vi "Car Wash Main.vi"(0 "Deluxe Wash":bool, 7 "Economy wash":bool, 9 "stop":bool, 11 "Error in":errorcluster) -> (4 "Under body wash":bool, 6 "Soap application":bool, 8 "Main high pressure wash":bool, 10 "Clear water rinse":bool, 15 "error out":errorcluster)   [LabVIEW 2020, in "Car Wash.lvlib"]
doc: "This system is a state machine of car wash system which has two different modes for users such as premium and genric car wash"
uses:
  Car Wash.lvlib
  Typedefs/Queue operations.ctl
  Typedefs/Car wash data.ctl
panel:
  out "Elapsed Time":dbl
  out "Vehicle out of position":bool
  out "Air dry":bool
  in  "Air dry\nposition\nswitch":bool
  in  "Main wash\nPosition \nswitch":bool
  in  "Under Body\nWash Position \nswitch":bool
  # "Purchase Section"
  # "Car Wash Simulators"
  # "Car Wash Simulation Switches"
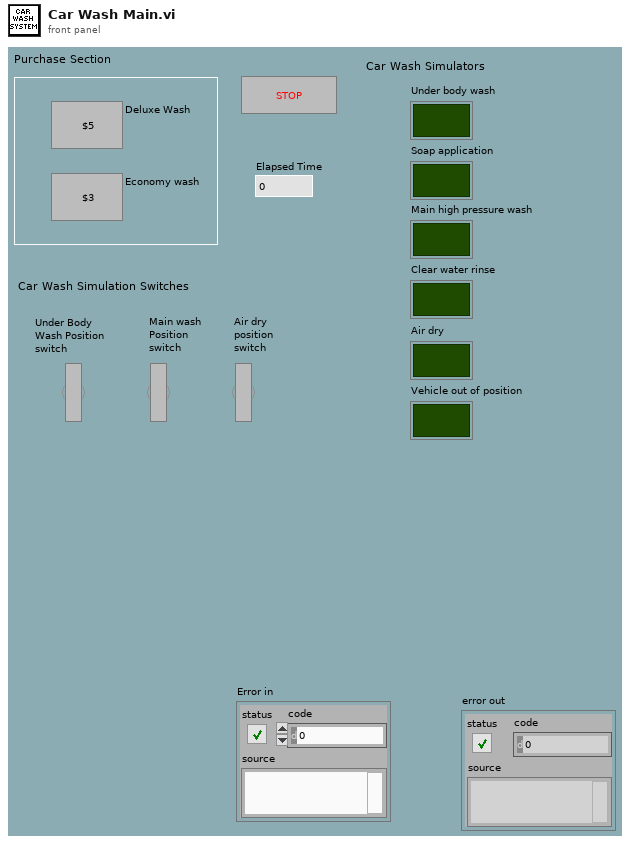
[diagram p1: front panel]
types:
  T1 = typedef "Car wash data.ctl" = cluster{"Start Time":timestamp, "Elapsed Time":dbl, "Set Time":dbl, "Previous Time":dbl, "Started?":bool, "Paused?":bool, "Enable controls ref":refnum<vi>[], "Disable controls ref":refnum<vi>[], "Soap application":bool, "Main high pressure wash":bool, "Under body wash":bool, "Clean water wash":bool, "Air dry":bool, "Vehicle out of position":bool, "Deluxe":bool, "Economy":bool, "Stop":bool}
  T2 = typedef "Car Wash.lvlib/Queue operations.ctl" = enum16{"Create queue", "Enqueue", "Enstack", "Dequeue", "Flush queue", "Release queue"}
  T3 = enum8{"Enabled", "Disabled", "Disabled and Grayed Out"}
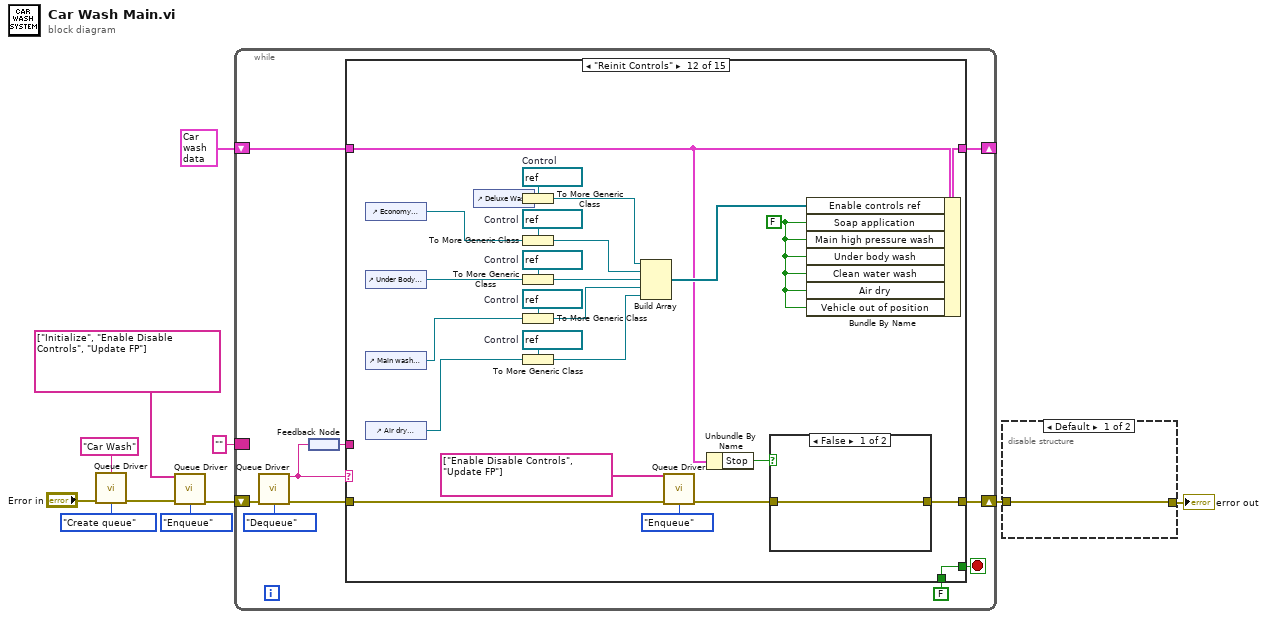
[diagram p0: block diagram]
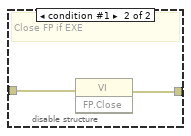
[diagram p2: hidden frame]
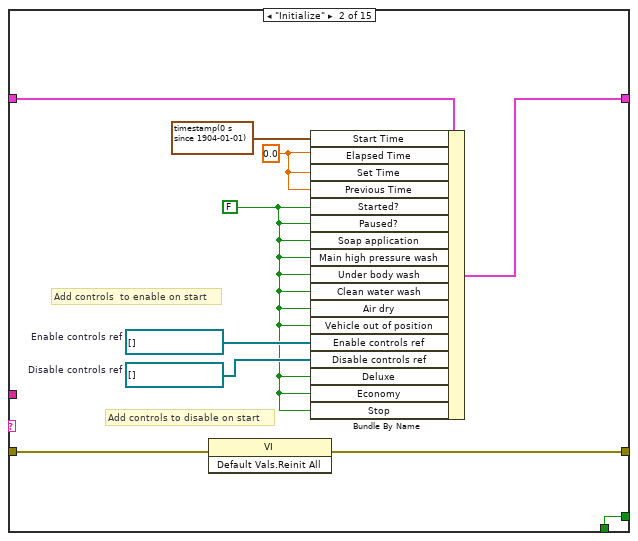
[diagram p4: hidden frame]
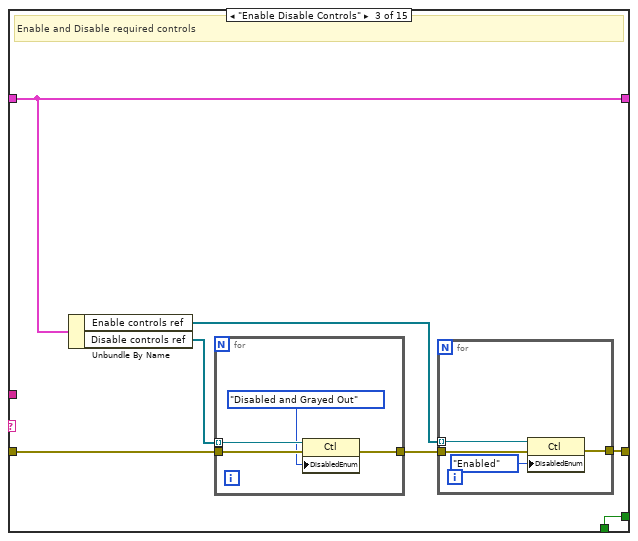
[diagram p5: hidden frame]
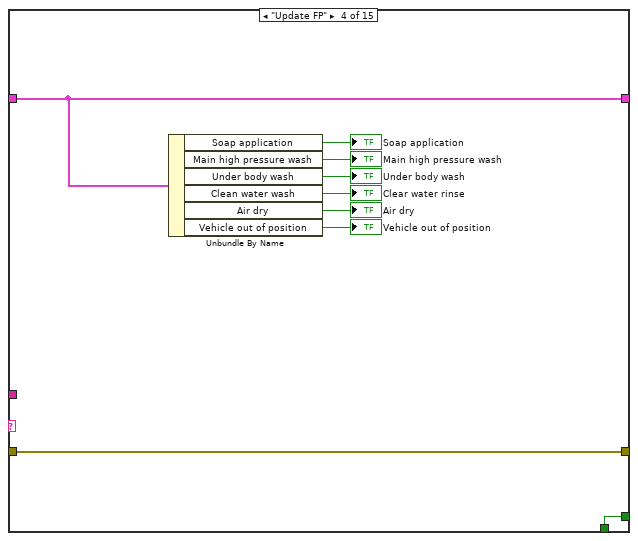
[diagram p6: hidden frame]
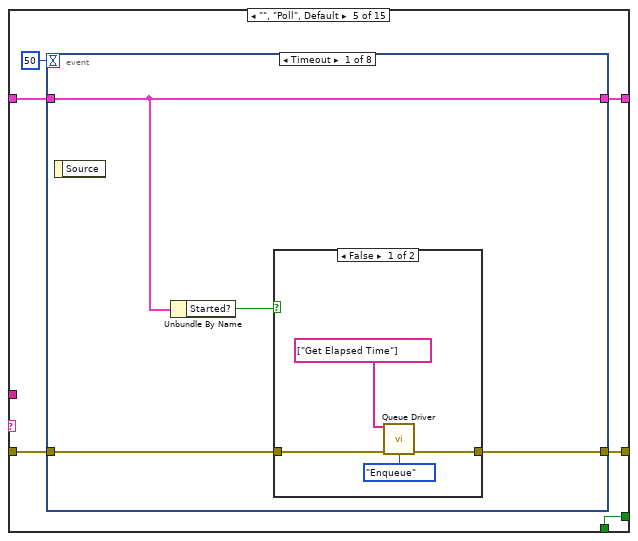
[diagram p7: hidden frame]
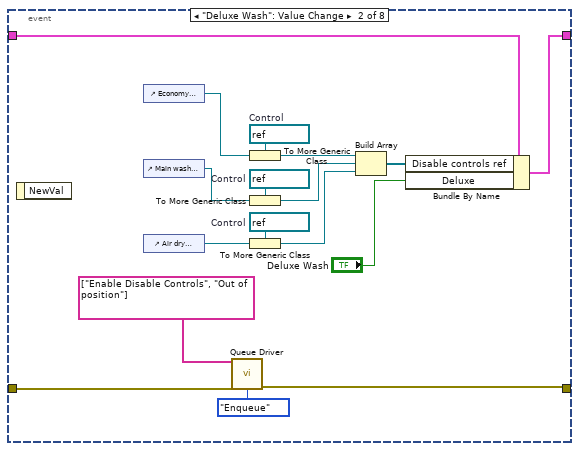
[diagram p9: hidden frame]
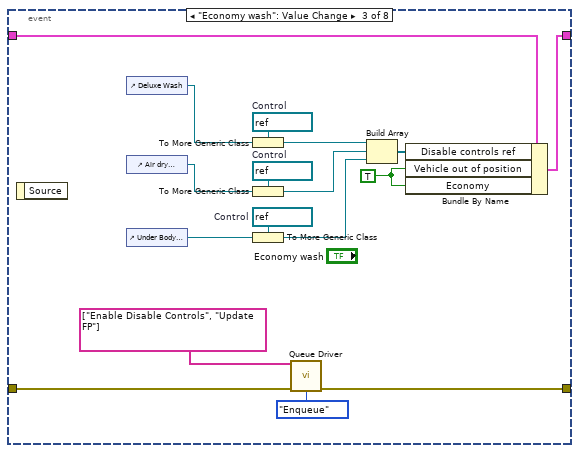
[diagram p10: hidden frame]
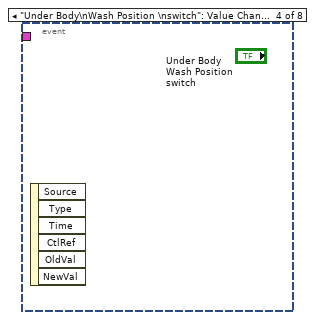
[diagram p11: hidden frame]
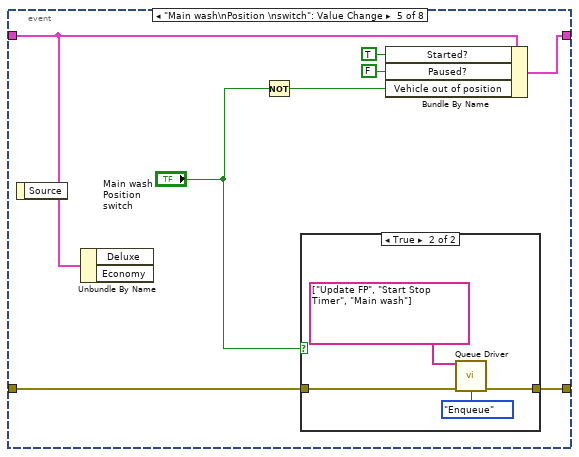
[diagram p12: hidden frame]
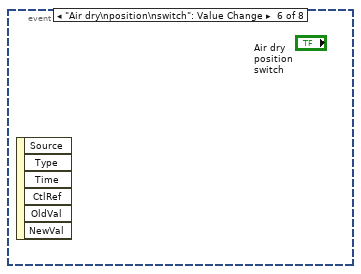
[diagram p14: hidden frame]
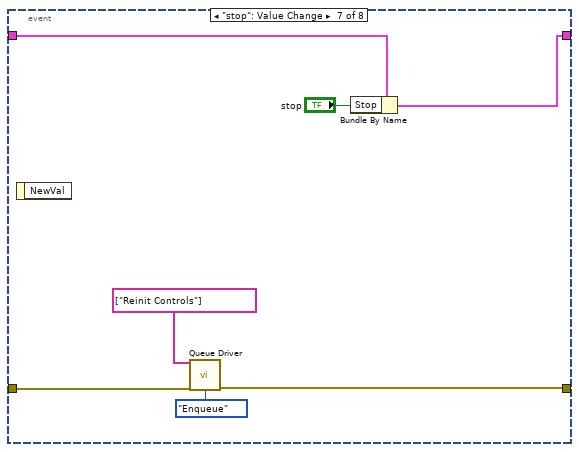
[diagram p15: hidden frame]
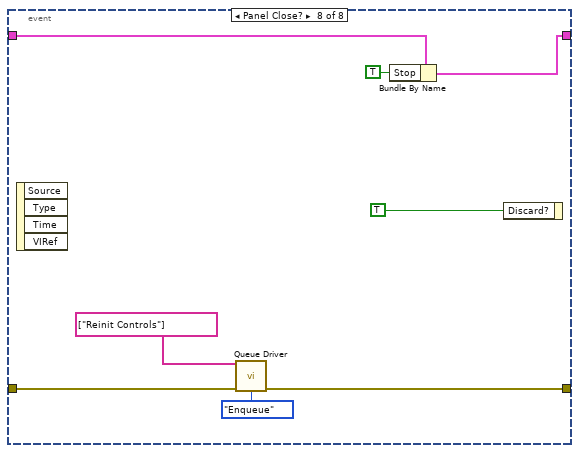
[diagram p16: hidden frame]
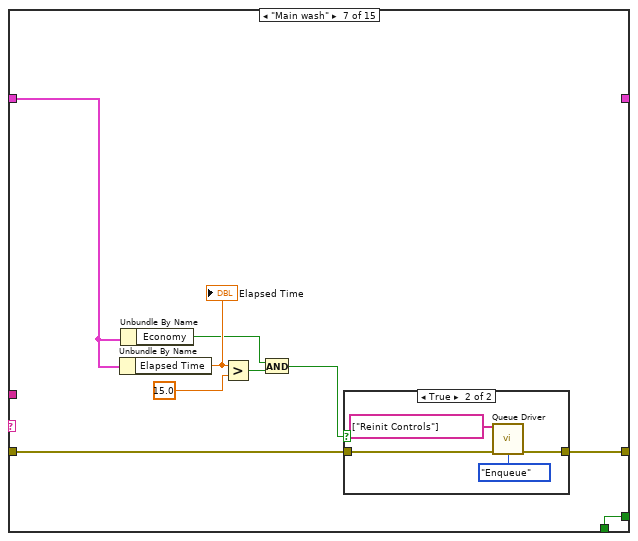
[diagram p18: hidden frame]
diagram:
  n1 = call "Queue Driver.vi"("Name"="Car Wash", "Error in"="Error in", "Operation"=Queue_operations."Create queue") -> ("Error out"=w10:errorcluster)  [unwired: 11 in, 1 out]
  n2 = call "Queue Driver.vi"("States"=string[] ["Initialize", "Enable Disable Controls", "Update FP"], "Error in"=w10, "Operation"=Queue_operations."Enqueue") -> ("Error out"=w5:errorcluster)  [unwired: 11 in, 1 out]
  n3 = while {
    border: "" ("Dequeued State") -> [_]
    shift-right: [w16] -> w3
    shift-left: w5 -> [w21]
    shift-right: [w14] -> _
    shift-left: T1 {"Start Time"=timestamp(0 s since 1904-01-01), "Elapsed Time"=0.0, "Set Time"=0.0, "Previous Time"=0.0, "Started?"=FALSE, "Paused?"=FALSE, "Enable controls ref"=[], "Disable controls ref"=[], "Soap application"=FALSE, "Main high pressure wash"=FALSE, "Under body wash"=FALSE, "Clean water wash"=FALSE, "Air dry"=FALSE, "Vehicle out of position"=FALSE, "Deluxe"=FALSE, "Economy"=FALSE, "Stop"=FALSE} -> [w15]
    stop <- w12 stop-if-true
    n4 = call "Queue Driver.vi"("Error in"=w21, "Operation"=Queue_operations."Dequeue") -> ("Dequeued State"=w19:string, "Error out"=w17:errorcluster)  [unwired: 12 in]
    n5 = feedback-in #1(w19) -> ()
    n6 = feedback #1() -> (w18:string)
    n7 = case shown="\"Reinit Controls\"" w19 {
      tunnel: w18 -> [_ _ _ _ _ _ _ _ _ _ _ _ _ w230 _]
      tunnel: [w23 w29 w37 w50 w60 w136 w139 w152 w154 w159 w164 w175 w204 w227 w249] -> w16
      tunnel: w17 -> [w23 w30 w39 w50 w61 w136 w140 w152 w154 w159 w164 w185 w205 w231 w247]
      tunnel: w15 -> [w24 w34 w41 w58 w62 _ w142 _ _ w157 w167 w174 w210 w226 w246]
      tunnel: [w24 w31 w41 w58 w63 _ _ _ _ w161 w166 w178 w209 w226 w246] -> w14
      tunnel: FALSE -> [w22 w26 w35 w51 w59 w137 w146 w153 w155 w160 w165 w184 w203 w225 _]
      tunnel: [w22 w26 w35 w51 w59 w137 w146 w153 w155 w160 w165 w184 w203 w225 TRUE] -> w12
      frame "/***Initialize***/" {
      }
      frame "Initialize" {
        w27 = refnum<vi>[] []  # Disable controls ref
        w28 = refnum<vi>[] []  # Enable controls ref
        w25 = FALSE
        w32 = 0.0
        # "Add controls to disable on start"
        # "Add controls  to enable on start"
        n8 = invoke class="VI" method="Default Vals.Reinit All"(error in=w30) -> (error out=w29:errorcluster)  [unwired: 2 in, 2 out]
        n9 = Bundle By Name(cluster=w34, "Start Time"=timestamp(0 s since 1904-01-01), "Elapsed Time"=w32, "Set Time"=w32, "Previous Time"=w32, "Started?"=w25, "Paused?"=w25, "Soap application"=w25, "Main high pressure wash"=w25, "Under body wash"=w25, "Clean water wash"=w25, "Air dry"=w25, "Vehicle out of position"=w25, "Enable controls ref"=w28, "Disable controls ref"=w27, "Deluxe"=w25, "Economy"=w25, "Stop"=w25) -> (w31:T1)
      }
      frame "Enable Disable Controls" {
        # "Enable and Disable required controls"
        n10 = Unbundle By Name(w41) -> ("Enable controls ref"=w40:refnum<vi>[], "Disable controls ref"=w36:refnum<vi>[])
        n11 = for {
          tunnel: w39 -> [w49]
          tunnel: [w48] -> w38
          tunnel: w36 -> [w47] mode=indexing
          n12 = property class="Ctl"(reference=w47, error in=w49, "DisabledEnum"=T3."Disabled and Grayed Out" ("Disabled")) -> (error out=w48:errorcluster)  [unwired: 1 out]
        }
        n13 = for {
          tunnel: w40 -> [w45] mode=indexing
          tunnel: w38 -> [w44]
          tunnel: [w42] -> w37
          n14 = property class="Ctl"(reference=w45, error in=w44, "DisabledEnum"=T3."Enabled" ("Disabled")) -> (error out=w42:errorcluster)  [unwired: 1 out]
        }
      }
      frame "Update FP" {
        n15 = Unbundle By Name(w58) -> ("Soap application"=→"Soap application":bool, "Main high pressure wash"=→"Main high pressure wash":bool, "Under body wash"=→"Under body wash":bool, "Clean water wash"=→"Clear water rinse":bool, "Air dry"=→"Air dry":bool, "Vehicle out of position"=→"Vehicle out of position":bool)
      }
      frame "", "Poll", Default {
        n16 = event shown="[0] Timeout" {
          selector: _ -> [_ _ _ _ _ _ _ _]
          dyn-events: _ -> [_ _ _ _ _ _ _ _]
          timeout: 50 -> [_ _ _ _ _ _ _ _]
          tunnel: [w68 w89 w106 _ w112 _ w122 w129] -> w63
          tunnel: w62 -> [w68 w90 w107 _ w113 _ w123 w130]
          tunnel: w61 -> [w67 w87 w102 _ w115 _ w127 w132]
          tunnel: [w66 w86 w101 _ w114 _ w126 w131] -> w60
          event Timeout {
            n17 = event-data() -> ()  [unwired: 1 in, 1 out]
            n18 = Unbundle By Name(w68) -> ("Started?"=w65:bool)
            n19 = case shown="False" w65 {
              tunnel: w67 -> [w72 w73]
              tunnel: [w71 w73] -> w66
              frame False {
                n20 = call "Queue Driver.vi"("States"=string[] ["Get Elapsed Time"], "Error in"=w72, "Operation"=Queue_operations."Enqueue") -> ("Error out"=w71:errorcluster)  [unwired: 11 in, 1 out]
              }
              frame True {
              }
            }
          }
          event "Deluxe Wash": Value Change {
            w79 = refnum<vi> refnum  # Control
            w80 = refnum<vi> refnum  # Control
            w82 = refnum<vi> refnum  # Control
            n21 = event-data() -> ()  [unwired: 1 in, 1 out]
            n22 = control-ref of="Economy wash"() -> (w83:refnum<vi>)
            n23 = control-ref of="Main wash\nPosition \nswitch"() -> (w77:refnum<vi>)
            n24 = control-ref of="Air dry\nposition\nswitch"() -> (w78:refnum<vi>)
            n25 = call "Queue Driver.vi"("States"=string[] ["Enable Disable Controls", "Out of position"], "Error in"=w87, "Operation"=Queue_operations."Enqueue") -> ("Error out"=w86:errorcluster)  [unwired: 11 in, 1 out]
            n26 = To More Generic Class(target class=w82, reference=w83) -> (generic class reference=w81:refnum<vi>)
            n27 = To More Generic Class(target class=w80, reference=w77) -> (generic class reference=w76:refnum<vi>)
            n28 = To More Generic Class(target class=w79, reference=w78) -> (generic class reference=w75:refnum<vi>)
            n29 = Build Array(w81, w76, w75) -> (w88:refnum<vi>[])
            n30 = Bundle By Name(cluster=w90, "Disable controls ref"=w88, "Deluxe"="Deluxe Wash") -> (w89:T1)
          }
          event "Economy wash": Value Change {
            w91 = TRUE ("Vehicle out of position")
            w96 = refnum<vi> refnum  # Control
            w97 = refnum<vi> refnum  # Control
            w98 = refnum<vi> refnum  # Control
            n31 = event-data() -> ()  [unwired: 1 in, 1 out]
            n32 = control-ref of="Deluxe Wash"() -> (w104:refnum<vi>)
            n33 = control-ref of="Air dry\nposition\nswitch"() -> (w92:refnum<vi>)
            n34 = control-ref of="Under Body\nWash Position \nswitch"() -> (w95:refnum<vi>)
            n35 = To More Generic Class(target class=w98, reference=w104) -> (generic class reference=w99:refnum<vi>)
            n36 = To More Generic Class(target class=w97, reference=w92) -> (generic class reference=w94:refnum<vi>)
            n37 = To More Generic Class(target class=w96, reference=w95) -> (generic class reference=w93:refnum<vi>)
            n38 = call "Queue Driver.vi"("States"=string[] ["Enable Disable Controls", "Update FP"], "Error in"=w102, "Operation"=Queue_operations."Enqueue") -> ("Error out"=w101:errorcluster)  [unwired: 11 in, 1 out]
            n39 = Build Array(w99, w94, w93) -> (w105:refnum<vi>[])
            n40 = Bundle By Name(cluster=w107, "Disable controls ref"=w105, "Vehicle out of position"=w91, "Economy"=w91) -> (w106:T1)
          }
          event "Under Body\nWash Position \nswitch": Value Change {
            n41 = event-data() -> ()  [unwired: 1 in, 6 out]
          }
          event "Main wash\nPosition \nswitch": Value Change {
            n42 = event-data() -> ()  [unwired: 1 in, 1 out]
            n43 = Unbundle By Name(w113) -> ()  [unwired: 2 out]
            n44 = Not(x="Main wash\nPosition \nswitch") -> (.not. x?=w111:bool)
            n45 = case shown="True" "Main wash\nPosition \nswitch" {
              tunnel: w115 -> [w116 w119]
              tunnel: [w116 w118] -> w114
              frame False {
              }
              frame True {
                n46 = call "Queue Driver.vi"("States"=string[] ["Update FP", "Start Stop Timer", "Main wash"], "Error in"=w119, "Operation"=Queue_operations."Enqueue") -> ("Error out"=w118:errorcluster)  [unwired: 11 in, 1 out]
              }
            }
            n47 = Bundle By Name(cluster=w113, "Started?"=TRUE, "Paused?"=FALSE, "Vehicle out of position"=w111) -> (w112:T1)
          }
          event "Air dry\nposition\nswitch": Value Change {
            n48 = event-data() -> ()  [unwired: 1 in, 6 out]
          }
          event "stop": Value Change {
            n49 = event-data() -> ()  [unwired: 1 in, 1 out]
            n50 = call "Queue Driver.vi"("States"=string[] ["Reinit Controls"], "Error in"=w127, "Operation"=Queue_operations."Enqueue") -> ("Error out"=w126:errorcluster)  [unwired: 11 in, 1 out]
            n51 = Bundle By Name(cluster=w123, "Stop"="stop") -> (w122:T1)
          }
          event Panel Close? {
            n52 = event-data() -> ()  [unwired: 1 in, 4 out]
            n53 = call "Queue Driver.vi"("States"=string[] ["Reinit Controls"], "Error in"=w132, "Operation"=Queue_operations."Enqueue") -> ("Error out"=w131:errorcluster)  [unwired: 11 in, 1 out]
            n54 = Bundle By Name(cluster=w130, "Stop"=TRUE) -> (w129:T1)
            n55 = event-data("Discard?"=TRUE) -> ()  [unwired: 1 in, 1 out]
          }
        }
      }
      frame "Under body wash" {
      }
      frame "Main wash" {
        n56 = Unbundle By Name(w142) -> ("Elapsed Time"=w145:dbl)
        "Elapsed Time" <- w145
        n57 = Unbundle By Name(w142) -> ("Economy"=w141:bool)
        n58 = Greater?(x=w145, y=15.0) -> (0:w143:bool)
        n59 = And(x=w141, y=w143) -> (x .and. y?=w138:bool)
        n60 = case shown="True" w138 {
          tunnel: w140 -> [w147 w151]
          tunnel: [w147 w150] -> w139
          frame False {
          }
          frame True {
            n61 = call "Queue Driver.vi"("States"=string[] ["Reinit Controls"], "Error in"=w151, "Operation"=Queue_operations."Enqueue") -> ("Error out"=w150:errorcluster)  [unwired: 11 in, 1 out]
          }
        }
      }
      frame "Air dry" {
      }
      frame "Out of position" {
      }
      frame "Start Stop Timer" {
        w162 = 0.0
        n62 = Unbundle By Name(w157) -> ("Started?"=w156:bool)
        n63 = Get Date/Time In Seconds() -> (seconds since 1Jan1904=w163:timestamp)
        n64 = Bundle By Name(cluster=w157, "Start Time"=w163, "Elapsed Time"=w162, "Previous Time"=w162, "Started?"=w156, "Paused?"=FALSE) -> (w161:T1)
      }
      frame "Pause Resume Timer" {
        n65 = in-place {
          n66 = in-place-cluster #2(w167) -> ("Paused?"=w170:bool, "Elapsed Time"=w168:dbl)  [unwired: 2 out]
          n67 = Get Date/Time In Seconds() -> (seconds since 1Jan1904=w171:timestamp)
          n68 = Not(x=w170) -> (.not. x?=w169:bool)
          n69 = in-place-cluster #2("Start Time"=w171, "Paused?"=w169, "Elapsed Time"=w168, "Previous Time"=w168) -> (w166:T1)
        }
      }
      frame "Reinit Controls" {
        w172 = FALSE ("Soap application")
        w192 = refnum<vi> refnum  # Control
        w191 = refnum<vi> refnum  # Control
        w190 = refnum<vi> refnum  # Control
        w189 = refnum<vi> refnum  # Control
        w188 = refnum<vi> refnum  # Control
        n70 = control-ref of="Economy wash"() -> (w182:refnum<vi>)
        n71 = control-ref of="Under Body\nWash Position \nswitch"() -> (w181:refnum<vi>)
        n72 = control-ref of="Main wash\nPosition \nswitch"() -> (w180:refnum<vi>)
        n73 = control-ref of="Air dry\nposition\nswitch"() -> (w179:refnum<vi>)
        n74 = control-ref of="Deluxe Wash"() -> (w183:refnum<vi>)
        n75 = To More Generic Class(target class=w188, reference=w183) -> (generic class reference=w197:refnum<vi>)
        n76 = To More Generic Class(target class=w189, reference=w182) -> (generic class reference=w196:refnum<vi>)
        n77 = To More Generic Class(target class=w190, reference=w181) -> (generic class reference=w195:refnum<vi>)
        n78 = To More Generic Class(target class=w191, reference=w180) -> (generic class reference=w194:refnum<vi>)
        n79 = To More Generic Class(target class=w192, reference=w179) -> (generic class reference=w193:refnum<vi>)
        n80 = Build Array(w197, w196, w195, w194, w193) -> (w177:refnum<vi>[])
        n81 = call "Queue Driver.vi"("States"=string[] ["Enable Disable Controls", "Update FP"], "Error in"=w185, "Operation"=Queue_operations."Enqueue") -> ("Error out"=w176:errorcluster)  [unwired: 11 in, 1 out]
        n82 = Unbundle By Name(w174) -> ("Stop"=w173:bool)
        n83 = case shown="False" w173 {
          tunnel: w176 -> [w198 w202]
          tunnel: [w198 w201] -> w175
          frame False {
          }
          frame True {
            n84 = call "Queue Driver.vi"("States"=string[] ["Exit"], "Error in"=w202, "Operation"=Queue_operations."Enqueue") -> ("Error out"=w201:errorcluster)  [unwired: 11 in, 1 out]
          }
        }
        n85 = Bundle By Name(cluster=w174, "Enable controls ref"=w177, "Soap application"=w172, "Main high pressure wash"=w172, "Under body wash"=w172, "Clean water wash"=w172, "Air dry"=w172, "Vehicle out of position"=w172) -> (w178:T1)
      }
      frame "Get Elapsed Time" {
        # "Elapsed Time = Current time - Start Time + Previous time"
        n86 = Unbundle By Name(w210) -> ("Start Time"=w212:timestamp, "Paused?"=w213:bool, "Previous Time"=w211:dbl, "Set Time"=w208:dbl)
        n87 = case shown="False" w213 {
          tunnel: w212 -> [w222 _]
          tunnel: w211 -> [w221 w224]
          tunnel: [w219 w224] -> w207
          frame False {
            n88 = Get Date/Time In Seconds() -> (seconds since 1Jan1904=w223:timestamp)
            n89 = Subtract(x=w223, y=w222) -> (x-y=w220:dbl)
            n90 = Add(x=w220, y=w221) -> (x+y=w219:dbl)
          }
          frame True {
          }
        }
        n91 = Less?(x=w207, y=w208) -> (x < y?=w206:bool)
        n92 = Bundle By Name(cluster=w210, "Elapsed Time"=w207) -> (w209:T1)
        n93 = case shown="False" w206 {
          tunnel: w205 -> [w214 w218]
          tunnel: [w214 w217] -> w204
          frame False {
          }
          frame True {
            n94 = call "Queue Driver.vi"("States"=string[] ["Start Stop Timer"], "Error in"=w218, "Operation"=Queue_operations."Dequeue") -> ("Error out"=w217:errorcluster)  [unwired: 11 in, 1 out]
          }
        }
      }
      frame "Error" {
        n95 = Unbundle By Name(w231) -> ("code"=w236:i32, "source"=w235:string)
        n96 = call <vilib>:"Clear Errors.vi"("error in (no error)"=w231, "specific error code to clear (0: all)"=w236) -> ("error out"=w238:errorcluster)  [unwired: 4 in, 1 out]
        n97 = Format Into String(format string="Error occurred in state \"%s\"!!\nError Code: %d\nError Source: %s\n\nDo you wish to continue?", error in=w238, w230, w236, w235) -> (resulting string=w234:string, error out=w229:errorcluster)  [unwired: 1 in]
        n98 = Two Button Dialog(message=w234, 1:"Exit" ("F button name (\"Cancel\")"), 2:"Continue" ("T button name (\"OK\")")) -> (T button?=w228:bool)
        n99 = case shown="False" w228 {
          tunnel: w229 -> [w244 w245]
          tunnel: [w241 w245] -> w227
          frame False {
            # "Exit"
            n100 = call "Queue Driver.vi"("Error in"=w244, "Operation"=Queue_operations."Flush queue") -> ("Error out"=w242:errorcluster)  [unwired: 12 in, 1 out]
            n101 = call "Queue Driver.vi"("States"=string[] ["Enable Disable Controls", "Update FP", "Exit"], "Error in"=w242, "Operation"=Queue_operations."Enqueue") -> ("Error out"=w241:errorcluster)  [unwired: 11 in, 1 out]
          }
          frame True {
            # "Continue"
          }
        }
      }
      frame "Exit" {
        n102 = call "Queue Driver.vi"("Error in"=w247, "Operation"=Queue_operations."Flush queue") -> ("Error out"=w250:errorcluster)  [unwired: 12 in, 1 out]
        n103 = call "Queue Driver.vi"("Error in"=w250, "Operation"=Queue_operations."Flush queue") -> ("Error out"=w249:errorcluster)  [unwired: 12 in, 1 out]
      }
    }
  }
  n104 = disable-structure shown="Default" {
    disable-tunnel: w3 -> [w253 w255]
    disable-tunnel: [w253 w254] -> w2
    frame condition #0 (active) {
    }
    frame condition #1 {
      # "Close FP if EXE"
      n105 = invoke class="VI" method="FP.Close"(error in=w255) -> (error out=w254:errorcluster)  [unwired: 2 in, 2 out]
    }
  }
  "error out" <- w2
